vi "IsValidNode.vi"(9 "y":i32, 10 "x":i32, 11 "OccupancyGridWorldMap in":refnum<class "NI_Robotics_OccupancyGridWorldMap.lvclass">) -> (2 "Valid":bool, 3 "OccupancyGridWorldMap out":refnum<class "NI_Robotics_OccupancyGridWorldMap.lvclass">)   [LabVIEW 2017, in "NI_Robotics_OccupancyGridWorldMap.lvclass"]
uses:
  <vilib>/robotics/Navigation/shared/WorldMap/OccupancyGridWorldMap/NI_Robotics_OccupancyGridWorldMap.lvclass
  <vilib>/robotics/Navigation/shared/WorldMap/OccupancyGridWorldMap/NI_Robotics_OccupancyGridWorldMap.lvclass/NI_Robotics_OccupancyGridWorldMap.ctl
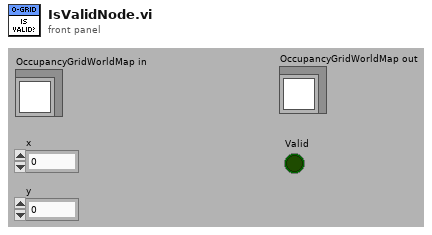
[diagram p1: front panel]
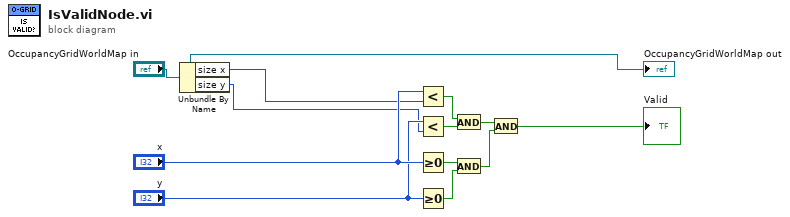
[diagram p0: block diagram]
diagram:
  n1 = Unbundle By Name("OccupancyGridWorldMap in") -> ("size x"=w3:i32, "size y"=w2:i32)
  n2 = Less?(x="x", y=w3) -> (x < y?=w6:bool)
  n3 = Less?(x="y", y=w2) -> (x < y?=w9:bool)
  n4 = Greater Or Equal To 0?(x="x") -> (x >= 0?=w8:bool)
  n5 = Greater Or Equal To 0?(x="y") -> (x >= 0?=w7:bool)
  n6 = And(x=w6, y=w9) -> (x .and. y?=w5:bool)
  n7 = And(x=w8, y=w7) -> (x .and. y?=w4:bool)
  n8 = And(x=w5, y=w4) -> (x .and. y?=→"Valid":bool)
  "OccupancyGridWorldMap out" <- "OccupancyGridWorldMap in"
